vi "sub_UDP_Init.vi"(11 "UDP Config":T1) -> (0 "error out":errorcluster, 2 "UDP Receiver session ID":refnum<k16>, 3 "UDP Transmitter session ID":refnum<k16>)   [LabVIEW 2012]
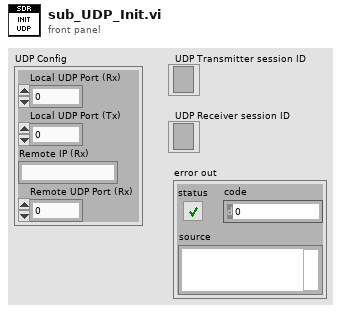
[diagram p1: front panel]
types:
  T1 = cluster{"Local UDP Port (Rx)":i16, "Local UDP Port (Tx)":i16, "Remote IP (Rx)":string, "Remote UDP Port (Rx)":i16}
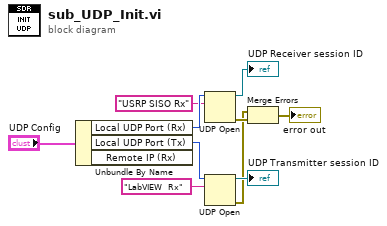
[diagram p0: block diagram]
diagram:
  n1 = Unbundle By Name("UDP Config") -> ("Local UDP Port (Rx)"=w5:i16, "Local UDP Port (Tx)"=w10:i16)  [unwired: 1 out]
  n2 = UDP Open(10:"USRP SISO Rx" ("service name"), 11:w5) -> (port=→"UDP Receiver session ID":refnum<k16>, 0:w7:errorcluster)  [unwired: 3 in, 1 out]
  n3 = UDP Open(10:"LabVIEW  Rx" ("service name"), 11:w10) -> (port=→"UDP Transmitter session ID":refnum<k16>, 0:w6:errorcluster)  [unwired: 3 in, 1 out]
  n4 = Merge Errors(w6, w7) -> (→"error out":errorcluster)
